vi "TSCAN Receive.vi"(0 "路径输入":path, 1 "读取报文类型":i8(ring) items=["只读取接收报文", "发送报文&接收报文"], 2 "BufferSize":i32=80, 3 "AAPPChannel":u32, 11 "错误输入（无错误）":errorcluster) -> (4 "路径输出":path, 14 "ACANMsgBuffer":T1(array[cluster]), 15 "错误输出":errorcluster)   [LabVIEW 2013]
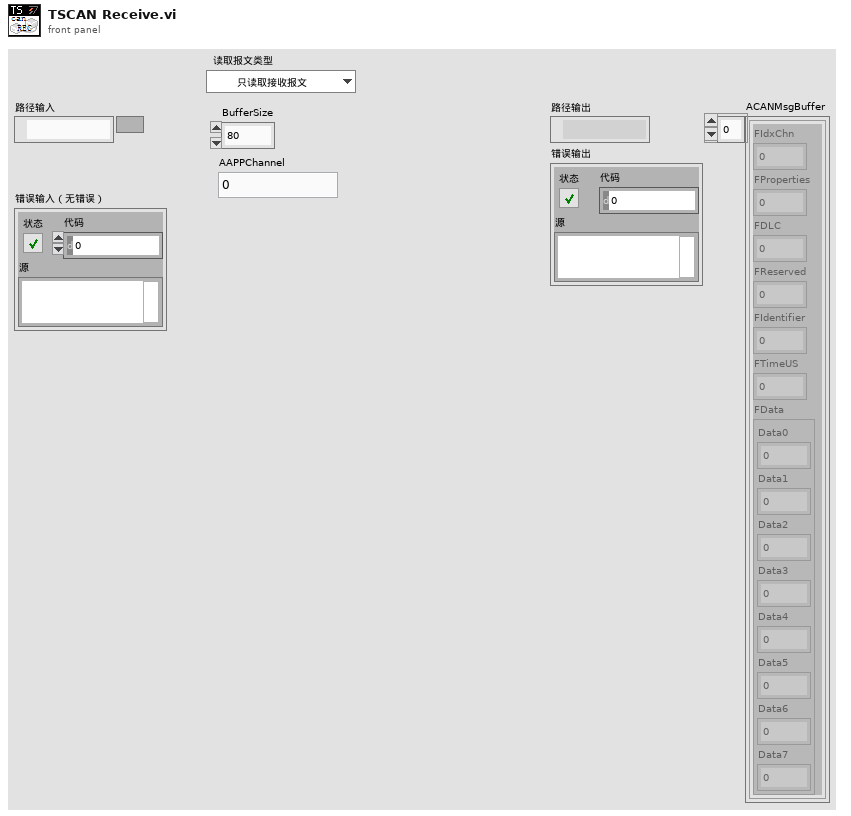
[diagram p1: front panel]
types:
  T1 = cluster{"FIdxChn":u8, "FProperties":u8, "FDLC":u8, "FReserved":u8, "FIdentifier":i32, "FTimeUS":u64, "FData":cluster{"Data0":u8, "Data1":u8, "Data2":u8, "Data3":u8, "Data4":u8, "Data5":u8, "Data6":u8, "Data7":u8}}[]
  T2 = cluster{"FIdxChn":u8, "FProperties":u8, "FDLC":u8, "FReserved":u8, "FIdentifier":i32, "FTimeUS":u64, "FData":cluster{"Data0":u8, "Data1":u8, "Data2":u8, "Data3":u8, "Data4":u8, "Data5":u8, "Data6":u8, "Data7":u8}}
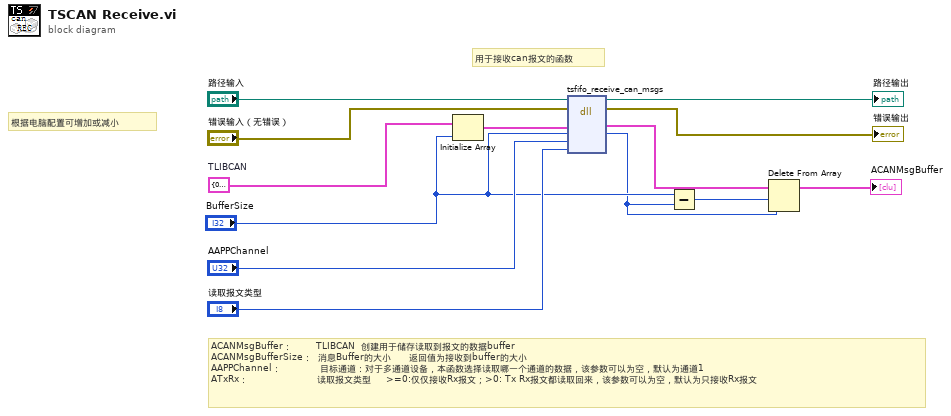
[diagram p0: block diagram]
diagram:
  w6 = T2 {"FIdxChn"=0, "FProperties"=0, "FDLC"=0, "FReserved"=0, "FIdentifier"=0, "FTimeUS"=0, "FData"={"Data0"=0, "Data1"=0, "Data2"=0, "Data3"=0, "Data4"=0, "Data5"=0, "Data6"=0, "Data7"=0}}  # TLIBCAN
  # "根据电脑配置可增加或减小"
  # "ACANMsgBuffer：        TLIBCAN  创建用于储存读取到报文的数据buffer\nACANMsgBufferSize：  消息Buffer的大小      返回值为接收到buffer的大小 \nAAPPChannel：             目标通道：对于多通道设备，本函数选择读取哪一个通道的数据，该参数可以为空，默认为通道1\nATxRx：                       读取报文类型     >=0:仅仅接收Rx报文；>0: Tx Rx报文都读取回来，该参数可以为空，默认为只接收Rx报文"
  # "用于接收can报文的函数"
  n1 = Initialize Array(w6, "BufferSize") -> (w13:T1)
  n2 = dll-call lib="PTH1Habs CUsers\nAdministratorDesktopTS_Can通讯PathTSMaster.dll" fn="tsfifo_receive_can_msgs"(path in="路径输入", error in="错误输入（无错误）", "ACANMsgBuffer"=w13, "ACANMsgBufferSize"="BufferSize", "AChn"="AAPPChannel", "ATxRx"="读取报文类型") -> (path out=→"路径输出":path, error out=→"错误输出":errorcluster, "ACANMsgBuffer"=w5:T1, "ACANMsgBufferSize"=w3:i32)  [unwired: 4 in]
  n3 = Subtract(x="BufferSize", y=w3) -> (x-y=w2:i32)
  n4 = Delete From Array(array=w5, length=w2, index=w3) -> (array with subset deleted=→"ACANMsgBuffer":T1)  [unwired: 1 out]
